vi "pickSurroundingPlatforms_TRAINING.vi"(10 "Goal \nplatform":i32, 11 "Start platform":i32) -> (3 "platform choices":i32[](array[numeric]))   [LabVIEW 2017]
panel:
  out "vector length":dbl
  out "distance of \nchoices":dbl[](array[numeric])
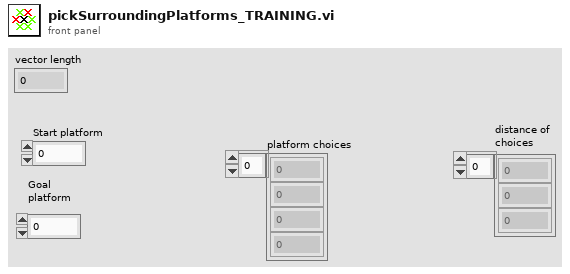
[diagram p1: front panel]
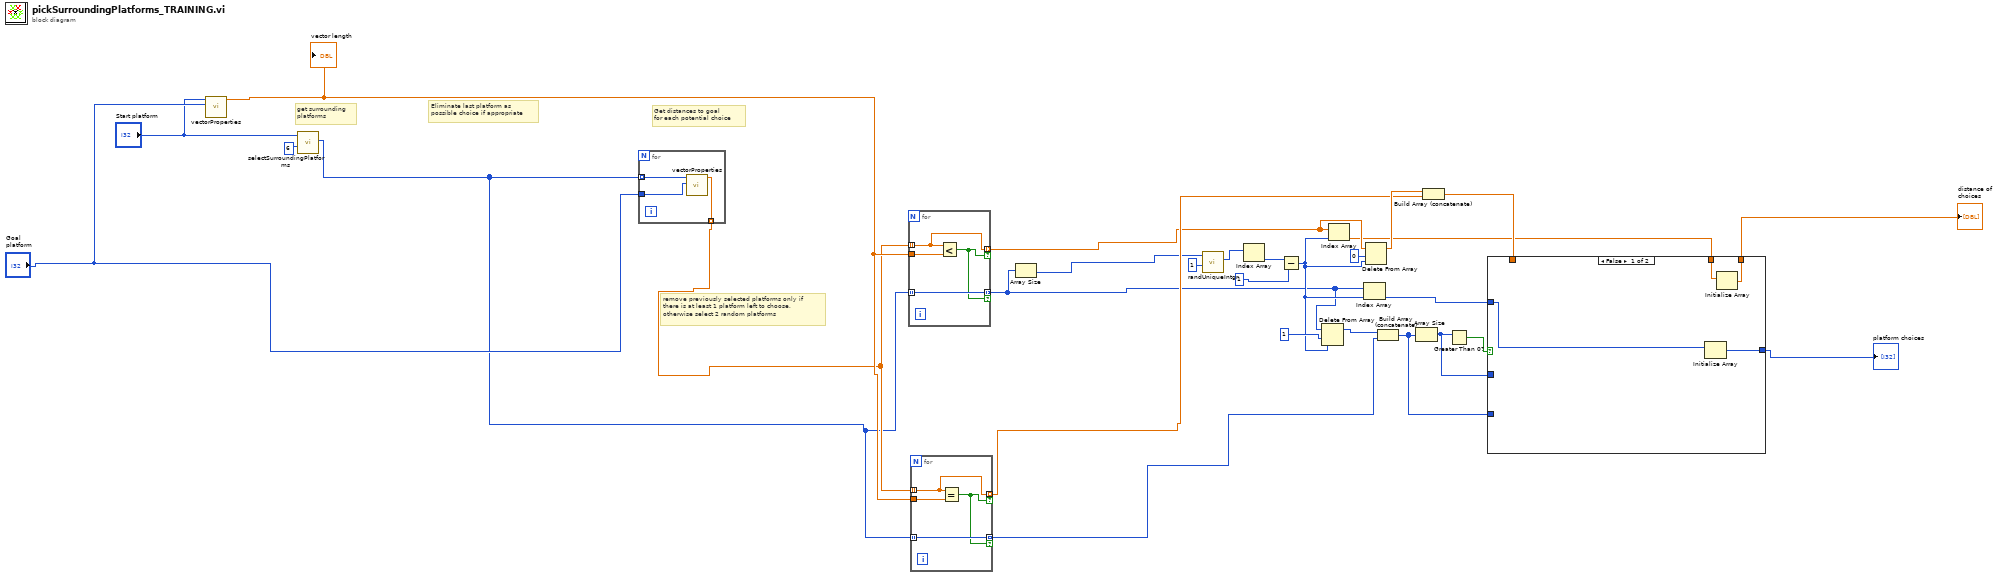
[diagram p0: block diagram]
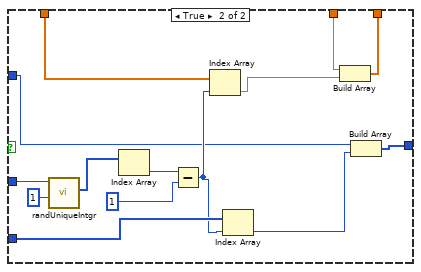
[diagram p2: hidden frame]
diagram:
  # "remove previously selected platforms only if \nthere is at least 1 platform left to choose,\notherwise select 2 random platforms"
  # "Get distances to goal\nfor each potential choice"
  # "Eliminate last platform as \npossible choice if appropriate"
  # "get surrounding\nplatforms"
  n1 = call "vectorProperties.vi"("Goal \nplatform"="Goal \nplatform", "Start \nplatform"="Start platform") -> ("vector length"=w25:dbl)  [unwired: 8 in, 1 out]
  "vector length" <- w25
  n2 = call "selectSurroundingPlatforms.vi"("Number of surrounding\nplatforms to raise"=6 ("Number of surrounding\nplatforms to raise"), "Start platform"="Start platform") -> ("Platforms \nto raise"=w1:i32[])  [unwired: 9 in]
  n3 = for {
    tunnel: "Goal \nplatform" -> [w31]
    tunnel: [w30] -> w2 mode=indexing
    tunnel: w1 -> [w29] mode=indexing
    n4 = call "vectorProperties.vi"("Goal \nplatform"=w31, "Start \nplatform"=w29) -> ("vector length"=w30:dbl)  [unwired: 8 in, 1 out]
  }
  n5 = for {
    tunnel: w2 -> [w32] mode=indexing
    tunnel: w25 -> [w35]
    tunnel: [w32] -> w7 mode=indexing if=w33
    tunnel: w1 -> [w34] mode=indexing
    tunnel: [w34] -> w9 mode=indexing if=w33
    n6 = Less?(x=w32, y=w35) -> (x < y?=w33:bool)
  }
  n7 = for {
    tunnel: w2 -> [w36] mode=indexing
    tunnel: w25 -> [w39]
    tunnel: [w36] -> w11 mode=indexing if=w37
    tunnel: w1 -> [w38] mode=indexing
    tunnel: [w38] -> w10 mode=indexing if=w37
    n8 = Equal?(x=w36, y=w39) -> (x = y?=w37:bool)
  }
  n9 = Array Size(array=w9) -> (size(s)=w8:i32)
  n10 = call "randUniqueIntgr.vi"("max rand number"=w8, "Number of Outputs"=1) -> ("output"=w22:u32[])  [unwired: 8 in]
  n11 = Index Array(array=w22) -> (element=w21:u32)  [unwired: 1 in]
  n12 = Subtract(x=w21, y=1) -> (x-y=w14:u32)
  n13 = Delete From Array(array=w9, length=1, index=w14) -> (array with subset deleted=w19:i32[])  [unwired: 1 out]
  n14 = Index Array(array=w7, index=w14) -> (element=w6:dbl)
  n15 = Index Array(array=w9, index=w14) -> (element=w4:i32)
  n16 = Delete From Array(array=w7, length=0, index=w14) -> (array with subset deleted=w13:dbl[])  [unwired: 1 out]
  n17 = Build Array (concatenate)(w19, w10) -> (w16:i32[])
  n18 = Array Size(array=w16) -> (size(s)=w17:i32)
  n19 = Build Array (concatenate)(w13, w11) -> (w12:dbl[])
  n20 = Greater Than 0?(x=w17) -> (x > 0?=w18:bool)
  n21 = case shown="False" w18 {
    tunnel: w17 -> [_ w56]
    tunnel: w16 -> [_ w52]
    tunnel: w12 -> [_ w51]
    tunnel: w6 -> [w42 w49]
    tunnel: [w43 w47] -> w5
    tunnel: w4 -> [w41 w46]
    tunnel: [w40 w44] -> w3
    frame False {
      n22 = Initialize Array(w41) -> (w40:i32[])  [unwired: 1 in]
      n23 = Initialize Array(w42) -> (w43:dbl[])  [unwired: 1 in]
    }
    frame True {
      n24 = call "randUniqueIntgr.vi"("max rand number"=w56, "Number of Outputs"=1) -> ("output"=w53:u32[])  [unwired: 8 in]
      n25 = Index Array(array=w53) -> (element=w55:u32)  [unwired: 1 in]
      n26 = Subtract(x=w55, y=1) -> (x-y=w50:u32)
      n27 = Index Array(array=w51, index=w50) -> (element=w48:dbl)
      n28 = Index Array(array=w52, index=w50) -> (element=w45:i32)
      n29 = Build Array(w49, w48) -> (w47:dbl[])
      n30 = Build Array(w46, w45) -> (w44:i32[])
    }
  }
  "platform choices" <- w3
  "distance of \nchoices" <- w5
